vi "zerncoeffs_RDgenerator.vi"(4 "Defocus":bool=TRUE, 6 "Tilts":bool=TRUE, 7 "idxType":enum16{"Wyant", "ANSI"}(ring)=enum."ANSI", 9 "Density":sgl=0.5 min=0 max=1 format="%#.4f", 10 "Aplitude":sgl=0.3 min=0 format="%#.4f", 11 "Max zern num":u32=14) -> (2 "Zern coeff":sgl[](array[numeric]), 3 "Zern index":i32[](array[numeric]))   [LabVIEW 2018]
uses:
  <vilib>/Analysis/1siggen.llb/Ramp Pattern by Delta.vi
  <vilib>/Analysis/NI_AALBase.lvlib
panel:
  # "Generate random Zernike coefficients"
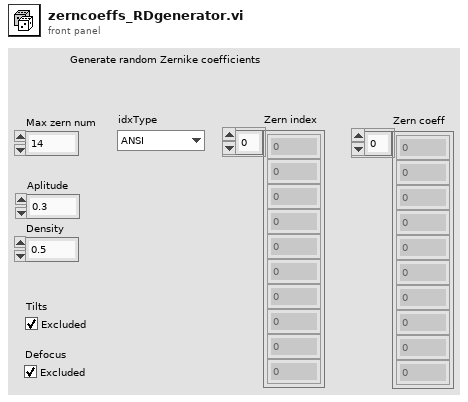
[diagram p1: front panel]
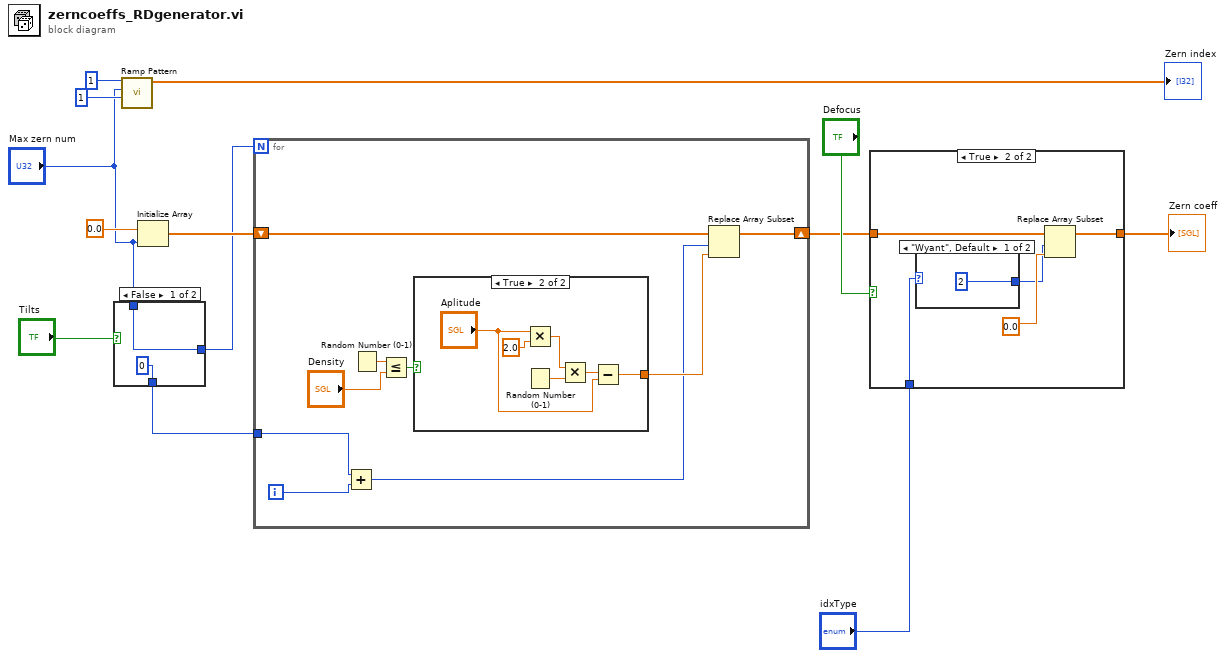
[diagram p0: block diagram]
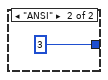
[diagram p3: hidden frame]
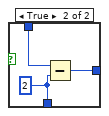
[diagram p4: hidden frame]
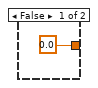
[diagram p5: hidden frame]
diagram:
  n1 = case shown="False" "Tilts" {
    tunnel: "Max zern num" -> [w15 w18]
    tunnel: [0 w16] -> w5
    tunnel: [w15 w17] -> w6
    frame False {
    }
    frame True {
      w16 = 2
      n2 = Subtract(x=w18, y=w16) -> (x-y=w17:u32)
    }
  }
  n3 = call-poly <vilib>:"Ramp Pattern.vi"("start"=1, "end"="Max zern num", "delta"=1) -> ("Ramp Pattern"=→"Zern index":dbl[])  [unwired: 6 in, 2 out]
  n4 = Initialize Array(sgl 0.0, "Max zern num") -> (w9:sgl[])
  n5 = for {
    N: w6 -> [_]
    shift-right: [w24] -> w3
    shift-left: w9 -> [w23]
    tunnel: w5 -> [w20]
    i -> [w21]
    n6 = Add(x=w20, y=w21) -> (x+y=w19:i32)
    n7 = Random Number (0-1)() -> (number: 0 to 1=w27:dbl)
    n8 = Less Or Equal?(x=w27, y="Density") -> (x <= y?=w26:bool)
    n9 = case shown="True" w26 {
      tunnel: [sgl 0.0 w31] -> w22
      frame False {
      }
      frame True {
        n10 = Multiply(x="Aplitude", y=2.0) -> (x*y=w34:dbl)
        n11 = Random Number (0-1)() -> (number: 0 to 1=w33:dbl)
        n12 = Multiply(x=w34, y=w33) -> (x*y=w32:dbl)
        n13 = Subtract(x=w32, y="Aplitude") -> (x-y=w31:dbl)
      }
    }
    n14 = Replace Array Subset(array=w23, new element=w22, index=w19) -> (w24:sgl[])
  }
  n15 = case shown="True" "Defocus" {
    tunnel: w3 -> [w35 w38]
    tunnel: [w35 w39] -> w2
    tunnel: "idxType" -> [_ w37]
    frame False {
    }
    frame True {
      n16 = case shown="\"Wyant\", Default" w37 {
        tunnel: [2 3] -> w36
        frame "Wyant", Default {
        }
        frame "ANSI" {
        }
      }
      n17 = Replace Array Subset(array=w38, new element=0.0, index=w36) -> (w39:sgl[])
    }
  }
  "Zern coeff" <- w2
